vi "Configure Sequence Trigger.vi"(0 "VISA resource name":refnum<visa-resource-name>, 1 "Trigger (0: Pattern 2 Entered)":u16(ring) items=["Pattern 2 Entered", " Pattern 2 Exited", "Edge 2", "Pattern 2 and Edge 2", "Nth Edge 2"], 11 "error in (no error)":errorcluster, 12 "Count (1)":i32=1) -> (4 "VISA resource name out":refnum<visa-resource-name>, 15 "error out":errorcluster)   [LabVIEW 2017, in "Agilent 6000 Series.lvlib"]
doc: "This VI configures the Sequence trigger. You specify the trigger and count with the Trigger and Count parameters.\n\n<B>NOTE:</B>\n\nThis VI is only valid for 6000 Series models. An error will be thrown if this VI is run with 5000 Series scopes."
uses:
  <instrlib>/Agilent 6000 Series/Agilent 6000 Series.lvlib
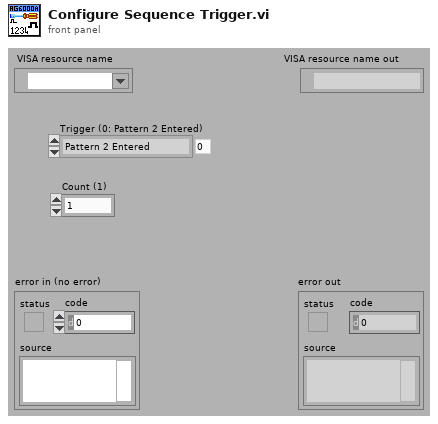
[diagram p1: front panel]
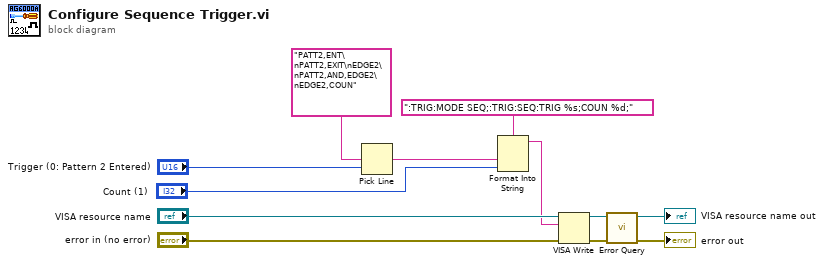
[diagram p0: block diagram]
diagram:
  n1 = Pick Line(multi-line string="PATT2,ENT\nPATT2,EXIT\nEDGE2\nPATT2,AND,EDGE2\nEDGE2,COUN", line index="Trigger (0: Pattern 2 Entered)") -> (output string=w3:string)  [unwired: 1 in]
  n2 = Format Into String(format string=":TRIG:MODE SEQ;:TRIG:SEQ:TRIG %s;COUN %d;" ("Source Command"), w3, "Count (1)") -> (resulting string=w5:string)  [unwired: 2 in, 1 out]
  n3 = VISA Write(VISA resource name="VISA resource name", write buffer=w5, error in (no error)="error in (no error)") -> (VISA resource name out=w8:refnum<visa-resource-name>, error out=w7:errorcluster)  [unwired: 1 out]
  n4 = call <instrlib>:"Error Query.vi"("error in (no error)"=w7, "VISA resource name"=w8) -> ("error out"=→"error out":errorcluster, "VISA resource name out"=→"VISA resource name out":refnum<visa-resource-name>)  [unwired: 6 in, 2 out]
